vi "svfa_Process Cross Power.vi"(0 "input signal X":waveform(dbl)={"t0"=timestamp(0 s since 1904-01-01), "dt"=1.953125e-05, "Y"=[]}, 1 "input signal Y":waveform(dbl)={"t0"=timestamp(0 s since 1904-01-01), "dt"=1.953125e-05, "Y"=[]}, 2 "window":T9=1 items=["None"=0, "Hanning"=1, "Hamming"=2, "Blackman-Harris"=3, "Exact Blackman"=4, "Blackman"=5, "Flat Top"=6, "4 Term B-Harris "=7, "7 Term B-Harris"=8, "Low Sidelobe"=9, "Force - Exponential"=10, "Blackman Nuttall"=11, "Triangle"=30, "Bartlett-Hanning"=31, "Bohman"=32, "Parzen"=33, "Welch"=34, "Kaiser"=60, "Dolph-Chebyshev"=61, "Gaussian"=62], 3 "force/exp settings":T7={"force window [%]"=50.0, "exponential window [%]"=10.0} {"exponential window [%]" min=0.0 max=100.0 format="%.2f"; "force window [%]" min=0.0 max=100.0 format="%.2f"}, 4 "averaging parameters":T11={"averaging mode"=enum."No averaging", "weighting mode"=enum."Linear", "number of averages"=10, "linear mode"=enum."Auto restart"}, 5 "error in (no error)":errorcluster, 7 "processing control in":T8(ring), 9 "spectrum info in":T1={"channel name"="", "description"="", "x-axis units"=0, "spectral info"={"spectrum type"=enum."Power [Magnitude^2]", "linear/dB"=enum."linear", "window"=0, "window size"=0, "FFT size"=0}, "engineering units"=0, "custom label"="", "dB reference [EU]"=0.0, "peak units"=enum."rms", "weighting filter"=0, "spectral density?"=FALSE, "unit label"="", "spectrum skewed?"=FALSE, "complimentary spectrum units"=enum."none"} {"x-axis units" items=["Time (s)"=0, "Frequency-CB (Hz)"=1, "Frequency-CPB (Hz)"=1248, "Frequency-Arbitrary (Hz)"=2357, "Quefrency (s)"=2, "Revolutions (rev)"=3, "Order"=4, "Speed (RPM)"=11, "Speed (rad/s)"=21, "Index"=65535]; "weighting filter" items=["Linear", "A-weighting", "B-weighting", "C-weighting", "ITU-R 468-4", "Dolby", "CCITT", "C-message", "Wb", "Wc", "Wd", "We", "Wf", "Wh", "Wj", "Wk", "Wm", "AES17 20 kHz lowpass", "AES17 40 kHz lowpass", "AES17 20 kHz highpass", "AES17 40 kHz highpass"]; "dB reference [EU]" format="%.2f"; "engineering units" items=["custom..."=0, "V"=1, "A"=21, "C"=30, "pC"=31, "s"=32, "-"=29, "Pa"=2, "N"=20, "g"=3, "m/s^2"=4, "m/s"=5, "m"=6, "mm/s"=12, "mm"=13, "micron/s"=14, "micron"=15, "in/s^2"=7, "in/s"=8, "in"=9, "mil/s"=10, "mil"=11, "rad/s^2"=16, "rad/s"=17, "rad"=18, "deg/s^2"=26, "deg/s"=27, "deg"=28, "RPM"=22, "cycle/s^2"=23, "Hz"=24, "cycle"=25, "strain"=19]; "spectral info"."window" items=["None "=0, "Hanning"=1, "Hamming"=2, "Blackman-Harris"=3, "Exact Blackman"=4, "Blackman"=5, "Flat Top"=6, "4 Term B-Harris "=7, "7 Term B-Harris"=8, "Low Sidelobe"=9, "Force - Exponential"=10, "Gaussian"=62]}) -> (12 "averages completed":dbl format="%.2f", 13 "processing control out":T8(ring), 14 "complex spectrum":T10={"f0"=0.0, "df"=1.0, "complex spectrum"=[]} {"complex spectrum" format="%.2f"; "df" format="%.2f"; "f0" format="%.2f"}, 17 "averaging done":bool, 18 "spectrum info out":T1={"channel name"="", "description"="", "x-axis units"=0, "spectral info"={"spectrum type"=enum."Power [Magnitude^2]", "linear/dB"=enum."linear", "window"=0, "window size"=0, "FFT size"=0}, "engineering units"=0, "custom label"="", "dB reference [EU]"=0.0, "peak units"=enum."rms", "weighting filter"=0, "spectral density?"=FALSE, "unit label"="", "spectrum skewed?"=FALSE, "complimentary spectrum units"=enum."none"} {"x-axis units" items=["Time (s)"=0, "Frequency-CB (Hz)"=1, "Frequency-CPB (Hz)"=1248, "Frequency-Arbitrary (Hz)"=2357, "Quefrency (s)"=2, "Revolutions (rev)"=3, "Order"=4, "Speed (RPM)"=11, "Speed (rad/s)"=21, "Index"=65535]; "weighting filter" items=["Linear", "A-weighting", "B-weighting", "C-weighting", "ITU-R 468-4", "Dolby", "CCITT", "C-message", "Wb", "Wc", "Wd", "We", "Wf", "Wh", "Wj", "Wk", "Wm", "AES17 20 kHz lowpass", "AES17 40 kHz lowpass", "AES17 20 kHz highpass", "AES17 40 kHz highpass"]; "dB reference [EU]" format="%.2f"; "engineering units" items=["custom..."=0, "V"=1, "A"=21, "C"=30, "pC"=31, "s"=32, "-"=29, "Pa"=2, "N"=20, "g"=3, "m/s^2"=4, "m/s"=5, "m"=6, "mm/s"=12, "mm"=13, "micron/s"=14, "micron"=15, "in/s^2"=7, "in/s"=8, "in"=9, "mil/s"=10, "mil"=11, "rad/s^2"=16, "rad/s"=17, "rad"=18, "deg/s^2"=26, "deg/s"=27, "deg"=28, "RPM"=22, "cycle/s^2"=23, "Hz"=24, "cycle"=25, "strain"=19]; "spectral info"."window" items=["None "=0, "Hanning"=1, "Hamming"=2, "Blackman-Harris"=3, "Exact Blackman"=4, "Blackman"=5, "Flat Top"=6, "4 Term B-Harris "=7, "7 Term B-Harris"=8, "Low Sidelobe"=9, "Force - Exponential"=10, "Gaussian"=62]}, 19 "error out":errorcluster)   [LabVIEW 2017]
uses:
  <vilib>/addons/_NISVFA/_Shared subVIs/Controls/svc_Window [Dual FFT].ctl
  <vilib>/addons/_NISVFA/_Shared subVIs/Controls/svc_Spectrum Info.ctl
  <vilib>/addons/_NISVFA/_Shared subVIs/Controls/svc_X-Axis Units.ctl
  <vilib>/addons/_NISVFA/_Shared subVIs/Controls/svc_Spectrum Type.ctl
  <vilib>/addons/_NISVFA/_Shared subVIs/Controls/svc_Engineering Units Text Ring.ctl
  <vilib>/addons/_NISVFA/_Shared subVIs/Controls/svc_Weighting Filter Text Ring.ctl
  <vilib>/addons/_NISVFA/_Shared subVIs/Controls/svc_Complimentary Spectrum Units.ctl
  <vilib>/addons/_NISVFA/_Shared subVIs/Windowing/svfa_Scaled Time Domain Window (1 Ch).vi
  <vilib>/addons/_NISVFA/_Shared subVIs/Spectrum Averaging/svfa_Reset Averaging State Info.vi
  <vilib>/addons/_NISVFA/_Shared subVIs/Spectrum Averaging/svfa_Average Array with Avg Checks (complex) No State.vi
  <vilib>/addons/_NISVFA/_Shared subVIs/Windowing/svfa_Scaled Time Domain Window (Array).vi
  <vilib>/addons/_NISVFA/_Shared subVIs/Spectrum Averaging/svfa_Average Array (complex) No State.vi
  <vilib>/Analysis/4window.llb/Force Window.vi
  <vilib>/Analysis/4window.llb/Force Window (DBL).vi
  <vilib>/Analysis/4window.llb/Exponential Window.vi
  <vilib>/Analysis/4window.llb/Exponential Window (DBL).vi
  <vilib>/addons/_NISVFA/_Shared subVIs/Spectrum Averaging/svfa_No Average Array (complex).vi
  <vilib>/addons/_NISVFA/_Shared subVIs/Spectrum Averaging/svfa_Average Array (complex).vi
  <vilib>/Utility/error.llb/Error Cluster From Error Code.vi
  <vilib>/Analysis/0measdsp.llb/Scaled Time Domain Window.vi
  <vilib>/Analysis/0measdsp.llb/Scaled Time Domain Window (DBL).vi
  <vilib>/addons/_NISVFA/_Spectrum Processing/subVIs/svfa_Spectrum Info Window to windowTd Type Def.vi
  <vilib>/addons/_NISVFA/_Shared subVIs/Common/svc_Window Parameters.vi
  <vilib>/addons/_NISVFA/_Shared subVIs/Common/svc_Get Window Info.vi
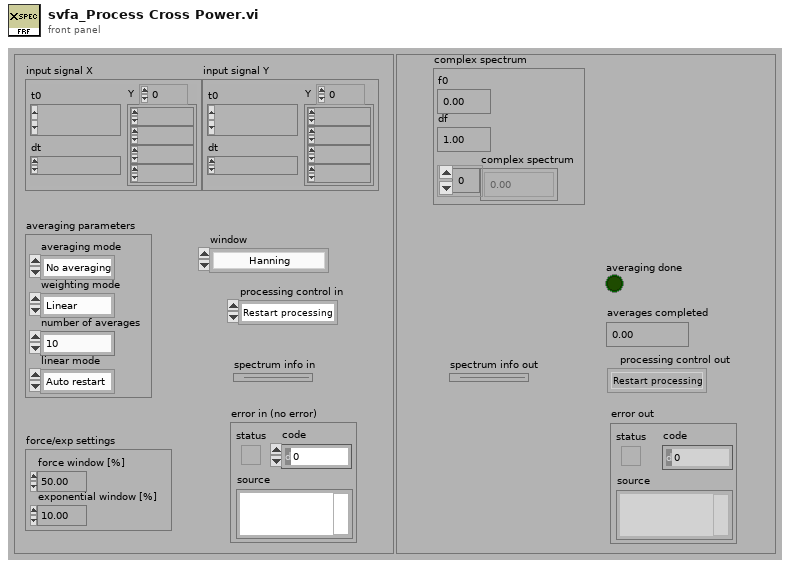
[diagram p1: front panel]
types:
  T1 = typedef "svc_Spectrum Info.ctl" = cluster{"channel name":string, "description":string, "x-axis units":T2, "spectral info":cluster{"spectrum type":T3, "linear/dB":enum16{"linear", "dB"}, "window":u16, "window size":i32, "FFT size":i32}, "engineering units":T4, "custom label":string, "dB reference [EU]":dbl, "peak units":enum16{"rms", "peak", "peak-peak"}, "weighting filter":T5, "spectral density?":bool, "unit label":string, "spectrum skewed?":bool, "complimentary spectrum units":T6}
  T2 = typedef "svc_X-Axis Units.ctl" = u16
  T3 = typedef "svc_Spectrum Type.ctl" = enum16{"FFT Spectrum [complex]", "Amplitude [Magnitude]", "Power [Magnitude^2]", "Cross Spectrum [complex]", "Frequency Response [Complex]"}
  T4 = typedef "svc_Engineering Units Text Ring.ctl" = u16
  T5 = typedef "svc_Weighting Filter Text Ring.ctl" = u16
  T6 = typedef "svc_Complimentary Spectrum Units.ctl" = enum16{"none", "radians", "degrees", "cycles", "imaginary"}
  T7 = cluster{"force window [%]":dbl, "exponential window [%]":dbl}
  T8 = enum16{"Restart processing", "Continue processing", "Skip processing"}
  T9 = typedef "svc_Window [Dual FFT].ctl" = u32
  T10 = cluster{"f0":dbl, "df":dbl, "complex spectrum":cdb[]}
  T11 = cluster{"averaging mode":enum16{"No averaging", "Vector averaging", "RMS averaging", "Peak hold"}, "weighting mode":enum16{"Linear", "Exponential"}, "number of averages":u32, "linear mode":enum16{"One shot", "Auto restart"}}
  T12 = enum16{"No averaging", "Vector averaging", "RMS averaging", "Peak hold"}
  T13 = cluster{"df":dbl, "df [Hz]":dbl, "average spectrum":cdb[]}
  T14 = cluster{"complex spectrum":cluster{"f0":dbl, "df":dbl, "complex spectrum":cdb[]}, "spectrum info":T1}
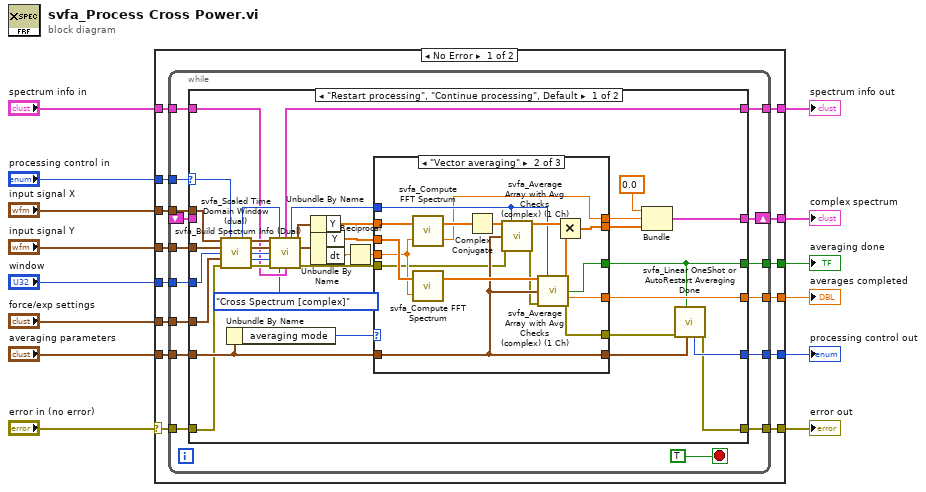
[diagram p0: block diagram]
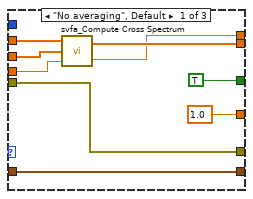
[diagram p2: hidden frame]
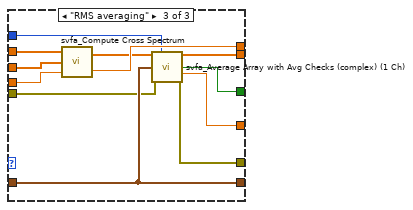
[diagram p3: hidden frame]
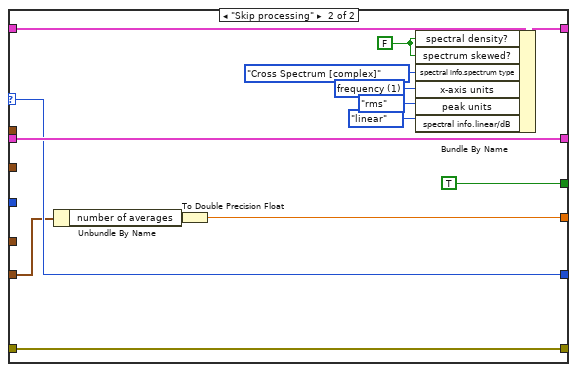
[diagram p4: hidden frame]
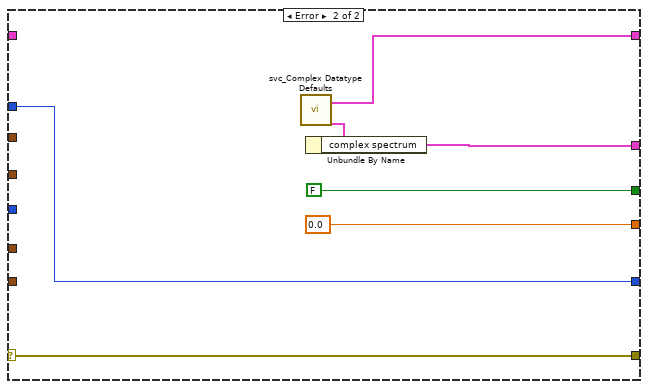
[diagram p5: hidden frame]
diagram:
  n1 = case shown="No Error" "error in (no error)" {
    selector: "error in (no error)" -> [w23 w138]
    tunnel: [w18 w138] -> w14
    tunnel: "averaging parameters" -> [w28 _]
    tunnel: "input signal X" -> [w26 _]
    tunnel: "input signal Y" -> [w25 _]
    tunnel: [w27 0.0 ("averages completed")] -> w10
    tunnel: [w22 FALSE ("averaging done")] -> w9
    tunnel: [w17 w132] -> w7
    tunnel: "processing control in" -> [w24 w135]
    tunnel: [w21 w135] -> w5
    tunnel: "window" -> [w20 _]
    tunnel: "force/exp settings" -> [w19 _]
    tunnel: [w16 w134] -> w2
    tunnel: "spectrum info in" -> [w15 _]
    frame No Error {
      n2 = while {
        shift-left: _ -> [w31]
        shift-right: [w32] -> w17
        tunnel: [w35] -> w18
        tunnel: w19 -> [w36]
        tunnel: w20 -> [w37]
        tunnel: [w38] -> w21
        tunnel: [w39] -> w22
        tunnel: w23 -> [w40]
        tunnel: w24 -> [w33]
        tunnel: w25 -> [w41]
        tunnel: w26 -> [w42]
        tunnel: [w43] -> w27
        tunnel: w28 -> [w44]
        tunnel: [w30] -> w16
        tunnel: w15 -> [w29]
        stop <- TRUE stop-if-true
        n3 = case shown="\"Restart processing\", \"Continue processing\", Default" w33 {
          selector: w33 -> [w60 w129]
          tunnel: w44 -> [w78 w127]
          tunnel: [w77 w125] -> w43
          tunnel: w42 -> [w76 _]
          tunnel: w41 -> [w73 _]
          tunnel: w40 -> [w72 w128]
          tunnel: [w69 TRUE ("averaging done")] -> w39
          tunnel: [w68 w129] -> w38
          tunnel: w37 -> [w67 _]
          tunnel: w36 -> [w66 _]
          tunnel: [w48 w131] -> w32
          tunnel: [w63 w128] -> w35
          tunnel: w31 -> [_ w131]
          tunnel: [w47 w118] -> w30
          tunnel: w29 -> [w46 w119]
          frame "Restart processing", "Continue processing", Default {
            n4 = call <vilib>:"svfa_Scaled Time Domain Window (dual).vi"("Signal in [X]"=w76, "processing control"=w60, "Signal in [Y]"=w73, "window"=w67, "force/exp settings"=w66, "error in (no error)"=w72) -> ("dup processing control"=w62:T8, "Windowed signal [X]"=w75:waveform(dbl), "Windowed signal [Y]"=w74:waveform(dbl), "window"=w64:T9, "window size"=w65:i32, "error out"=w71:errorcluster)  [unwired: 3 in, 1 out]
            n5 = Unbundle By Name(w78) -> ("averaging mode"=w79:T12)
            n6 = call <vilib>:"svfa_Build Spectrum Info (Dual).vi"("scaled signal  X [EU]"=w75, "processing control"=w62, "scaled signal  Y [EU]"=w74, "window"=w64, "window size"=w65, "error in (no error)"=w71, "spectrum type"=svc_Spectrum_Type."Cross Spectrum [complex]", "spectrum info in"=w46) -> ("spectrum info out"=w47:T1, "dup processing control"=w61:T8, "dup scaled signal  X [EU]"=w53:waveform(dbl), "dup scaled signal  Y [EU]"=w57:waveform(dbl), "error out"=w58:errorcluster)  [unwired: 3 in]
            n7 = Unbundle By Name ("Get Waveform Components")(w53) -> ("Y"=w54:dbl[])
            n8 = Unbundle By Name ("Get Waveform Components")(w57) -> ("Y"=w56:dbl[], "dt"=w55:dbl)
            n9 = Reciprocal(x=w55) -> (1/x=w50:dbl)
            n10 = case shown="\"Vector averaging\"" w79 {
              tunnel: w50 -> [w86 w101 w115]
              tunnel: w54 -> [w88 w103 w117]
              tunnel: w56 -> [w87 w102 w116]
              tunnel: w78 -> [w81 w94 w109]
              tunnel: w61 -> [_ w93 w110]
              tunnel: [w85 w100 w108] -> w49
              tunnel: [1.0 ("averages completed") w96 w111] -> w77
              tunnel: [TRUE ("averaging done") w95 w112] -> w69
              tunnel: [w84 w89 w114] -> w52
              tunnel: [w81 w94 w109] -> w70
              tunnel: w58 -> [w80 w92 w106]
              tunnel: [w80 w90 w107] -> w59
              frame "No averaging", Default {
                n11 = call <vilib>:"svfa_Compute Cross Spectrum.vi"("sampling frequency [Hz]"=w86, "signal Y [EUy]"=w87, "signal X [EUx]"=w88) -> ("df [Hz]"=w84:dbl, "cross spectrum [EUx EUy rms]"=w85:cdb[])
              }
              frame "Vector averaging" {
                n12 = call <vilib>:"svfa_Compute FFT Spectrum.vi"("sampling frequency [Hz]"=w101, "signal [EU]"=w103) -> ("df [Hz]"=w89:dbl, "FFT spectrum [EUrms]"=w104:cdb[])
                n13 = call <vilib>:"svfa_Compute FFT Spectrum.vi"("sampling frequency [Hz]"=w101, "signal [EU]"=w102) -> ("FFT spectrum [EUrms]"=w97:cdb[])  [unwired: 1 out]
                n14 = Complex Conjugate(1:w104) -> (0:w99:cdb[])
                n15 = call <vilib>:"svfa_Average Array with Avg Checks (complex) (1 Ch).vi"("spectrum"=w99, "processing control"=w93, "averaging parameters"=w94, "error in (no error)"=w92) -> ("average spectrum"=w98:cdb[], "error out"=w91:errorcluster)  [unwired: 7 in, 3 out]
                n16 = call <vilib>:"svfa_Average Array with Avg Checks (complex) (1 Ch).vi"("spectrum"=w97, "processing control"=w93, "averaging parameters"=w94, "error in (no error)"=w91) -> ("average spectrum"=w105:cdb[], "averaging done"=w95:bool, "averages completed"=w96:dbl, "error out"=w90:errorcluster)  [unwired: 7 in, 1 out]
                n17 = Multiply(x=w98, y=w105) -> (x*y=w100:cdb[])
              }
              frame "RMS averaging" {
                n18 = call <vilib>:"svfa_Compute Cross Spectrum.vi"("sampling frequency [Hz]"=w115, "signal Y [EUy]"=w116, "signal X [EUx]"=w117) -> ("df [Hz]"=w114:dbl, "cross spectrum [EUx EUy rms]"=w113:cdb[])
                n19 = call <vilib>:"svfa_Average Array with Avg Checks (complex) (1 Ch).vi"("spectrum"=w113, "processing control"=w110, "averaging parameters"=w109, "error in (no error)"=w106) -> ("average spectrum"=w108:cdb[], "averaging done"=w112:bool, "averages completed"=w111:dbl, "error out"=w107:errorcluster)  [unwired: 7 in, 1 out]
              }
            }
            n20 = Bundle("df"=0.0, "df [Hz]"=w52, "average spectrum"=w49) -> (w48:T13)  [unwired: 1 in]
            n21 = call <vilib>:"svfa_Linear OneShot or AutoRestart Averaging Done.vi"("averaging parameters"=w70, "averaging done"=w69, "error in (no error)"=w59) -> ("error out"=w63:errorcluster, "processing control"=w68:T8)  [unwired: 7 in]
          }
          frame "Skip processing" {
            w120 = u16 1 items=["time"=0, "frequency"=1, "quefrency"=2, "revolutions"=3, "order"=4, "rpm"=11] ("x-axis units")
            w122 = FALSE ("spectral density?")
            n22 = Unbundle By Name(w127) -> ("number of averages"=w126:u32)
            n23 = To Double Precision Float(number=w126) -> (double precision float=w125:dbl)
            n24 = Bundle By Name(cluster=w119, "spectral density?"=w122, "spectrum skewed?"=w122, "spectral info.spectrum type"=svc_Spectrum_Type."Cross Spectrum [complex]", "x-axis units"=w120, "peak units"=enum16{"rms", "peak", "peak-peak"}."rms", "spectral info.linear/dB"=enum16{"linear", "dB"}."linear") -> (w118:T1)
          }
        }
      }
    }
    frame Error {
      n25 = call <vilib>:"svc_Complex Datatype Defaults.vi"() -> ("dead spectrum info"=w134:T1, "complex spectrum"=w133:T14)  [unwired: 11 in, 7 out]
      n26 = Unbundle By Name(w133) -> ("complex spectrum"=w132:T10)
    }
  }
  "error out" <- w14
  "averages completed" <- w10
  "averaging done" <- w9
  "complex spectrum" <- w7
  "processing control out" <- w5
  "spectrum info out" <- w2
